vi "Analyse Board.vi"(8 "error in (no error)":errorcluster, 10 "GameBoard":u8[][](array[numeric]), 11 "CS++GoBangServer in":refnum<class "CS++GoBangServer.lvclass">) -> (0 "error out":errorcluster, 3 "CS++GoBangServer out":refnum<class "CS++GoBangServer.lvclass">)   [LabVIEW 2014, in "GoBang.lvlib" / "CS++GoBangServer.lvclass"]
uses:
  CS++GoBangServer.lvclass
  typdefs/GameState.ctl
  GoBang.lvlib
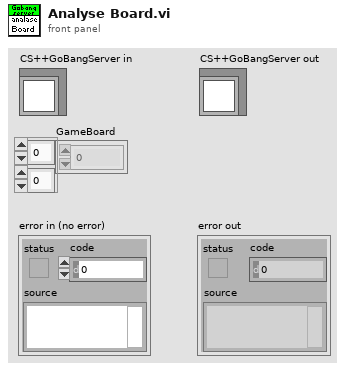
[diagram p1: front panel]
types:
  T1 = typedef "GoBang.lvlib/GameState.ctl" = enum16{"Waiting for opponent", "White to move", "Black to move", "Game over, white won", "Game over, black won"}
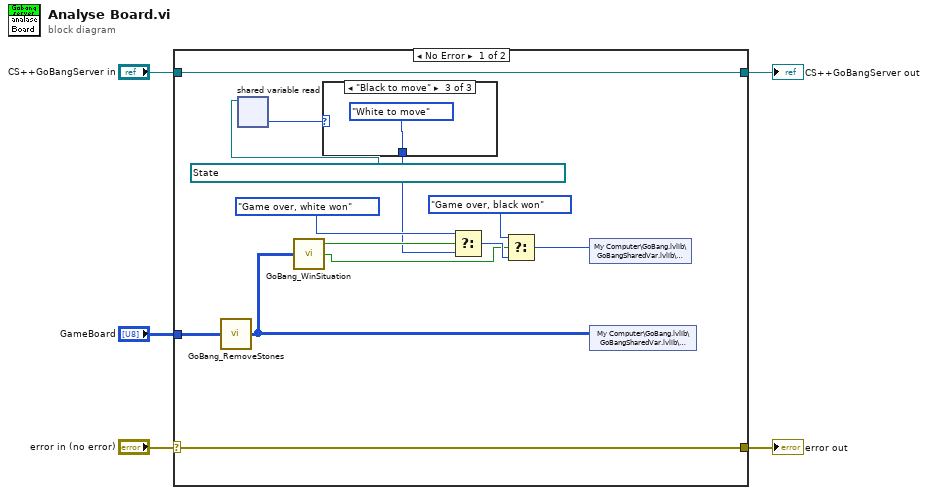
[diagram p0: block diagram]
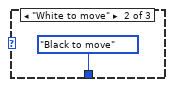
[diagram p3: hidden frame]
diagram:
  n1 = case shown="No Error" "error in (no error)" {
    selector: "error in (no error)" -> [w17 w23]
    tunnel: [w17 w23] -> w4
    tunnel: [w14 w22] -> w2
    tunnel: "CS++GoBangServer in" -> [w14 w22]
    tunnel: "GameBoard" -> [w18 _]
    frame No Error {
      w6 = refnum<k21> "ni.var.psp://My Computer/GoBang/GoBangSharedVar/GameState" items=["Waiting for opponent", "White to move", "Black to move", "Game over, white won", "Game over, black won"] ("shared variable refnum in")
      n2 = call "GoBang_RemoveStones.vi"("GameBoard in"=w18) -> ("GameBoard out"=w9:u8[][])
      n3 = shared-variable-read(w6) -> (w7:T1)  [unwired: 1 in, 2 out]
      n4 = call "GoBang_WinSituation.vi"("GameBoard"=w9) -> ("White won"=w16:bool, "Black won"=w12:bool)  [unwired: 1 out]
      n5 = case shown="\"Black to move\"" w7 {
        selector: w7 -> [w19 _ _]
        tunnel: [w19 GameState."Black to move" ("State") GameState."White to move" ("State")] -> w10
        frame "Waiting for opponent", Default {
        }
        frame "White to move" {
        }
        frame "Black to move" {
        }
      }
      n6 = Select(t=GameState."Game over, white won" ("State"), s=w16, f=w10) -> (s? t:f=w13:T1)
      n7 = Select(t=GameState."Game over, black won" ("State"), s=w12, f=w13) -> (s? t:f=w8:T1)
      n8 = shared-variable "My Computer\\GoBang.lvlib\\GoBangSharedVar.lvlib\\GameState"(w8) -> ()  [unwired: 1 in, 1 out]
      n9 = shared-variable "My Computer\\GoBang.lvlib\\GoBangSharedVar.lvlib\\GameBoard"(w9) -> ()  [unwired: 1 in, 1 out]
    }
    frame Error {
    }
  }
  "error out" <- w4
  "CS++GoBangServer out" <- w2
